vi "GetMeasured.vi"(8 "error in (no error)":errorcluster, 11 "Fake Code Coverage in":refnum<class "Fake Code Coverage.lvclass">) -> (0 "error out":errorcluster, 2 "All VIs Measured":path[](array[path]), 3 "Fake Code Coverage out":refnum<class "Fake Code Coverage.lvclass">)   [LabVIEW 2017, in "Cobertura.Tests.lvlib" / "Fake Code Coverage.lvclass"]
doc: "Returns the paths of all VIs for which code coverage data is available."
uses:
  Fake Code Coverage.lvclass
  Fake Code Coverage.lvclass/Fake Code Coverage.ctl
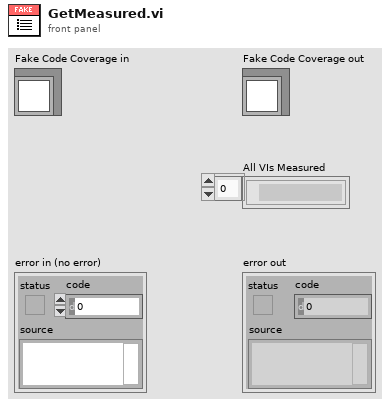
[diagram p1: front panel]
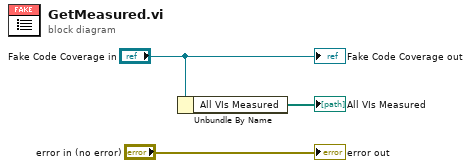
[diagram p0: block diagram]
diagram:
  n1 = Unbundle By Name("Fake Code Coverage in") -> ("All VIs Measured"=→"All VIs Measured":path[])
  "error out" <- "error in (no error)"
  "Fake Code Coverage out" <- "Fake Code Coverage in"
